vi "GlobalValue.vi"() -> ()   [LabVIEW 2020]
panel:
  in  "TempY":dbl
  in  "TempX":dbl
  in  "Y":dbl
  in  "X":dbl
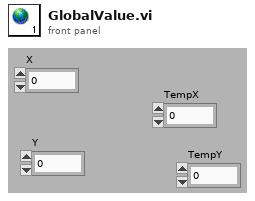
[diagram p1: front panel]
diagram:
